vi "CTIOTFInterfaceFGV.vi"(8 "error in":errorcluster, 10 "FGV_Control":u16(ring) items=["Set", "Get", "WaveformConvert"], 11 "data 2":refnum<visa-resource-name>) -> (0 "error out":errorcluster, 3 "data":refnum<visa-resource-name>)   [LabVIEW 2010]
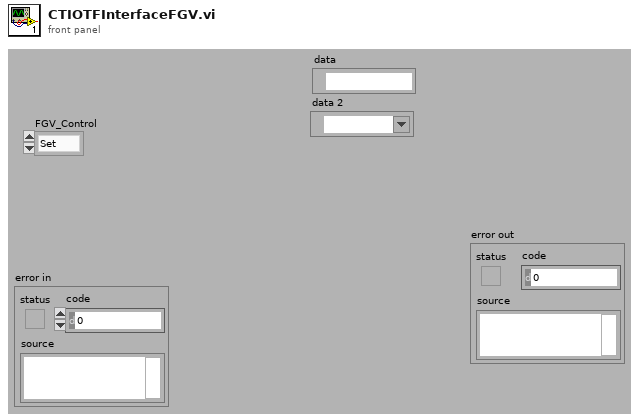
[diagram p1: front panel]
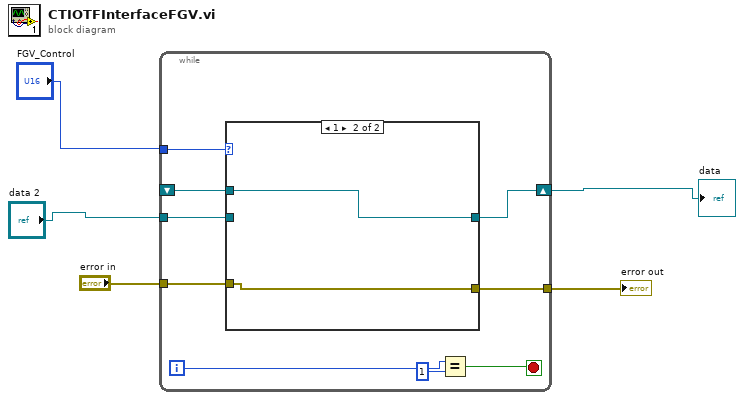
[diagram p0: block diagram]
diagram:
  n1 = while {
    tunnel: "FGV_Control" -> [w14]
    tunnel: "data 2" -> [w13]
    shift-right: [w12] -> w2
    shift-left: _ -> [w11]
    tunnel: [w7] -> w5
    tunnel: "error in" -> [w6]
    i -> [w9]
    stop <- w10 stop-if-true
    n2 = case shown="1" w14 {
      tunnel: w13 -> [w16 _]
      tunnel: [w16 w18] -> w12
      tunnel: w11 -> [_ w18]
      tunnel: [w15 w17] -> w7
      tunnel: w6 -> [w15 w17]
      frame 0, Default {
      }
      frame 1 {
      }
    }
    n3 = Equal?(x=w9, y=1) -> (x = y?=w10:bool)
  }
  "error out" <- w5
  "data" <- w2
